vi "Write Position.vi"(8 "error in":errorcluster, 10 "Position":bool, 11 "Switch Step in":refnum<class "Switch Step.lvclass">) -> (0 "error out":errorcluster, 3 "Switch Step out":refnum<class "Switch Step.lvclass">)   [LabVIEW 2012, in "Sequence Composition.lvlib" / "Switch Step.lvclass"]
uses:
  Switch Step.lvclass
  Switch Step.lvclass/Switch Step.ctl
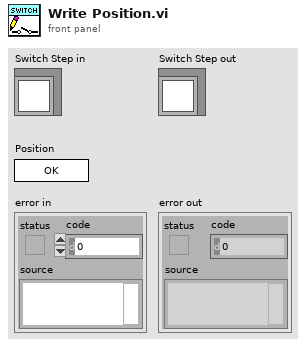
[diagram p1: front panel]
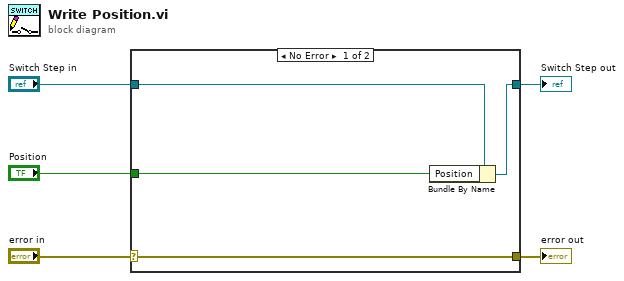
[diagram p0: block diagram]
diagram:
  n1 = case shown="No Error" "error in" {
    selector: "error in" -> [w9 w10]
    tunnel: [w9 w10] -> w4
    tunnel: [w7 w11] -> w2
    tunnel: "Switch Step in" -> [w8 w11]
    tunnel: "Position" -> [w6 _]
    frame No Error {
      n2 = Bundle By Name(cluster=w8, "Position"=w6) -> (w7:refnum<class "Switch Step.lvclass">)
    }
    frame Error {
    }
  }
  "error out" <- w4
  "Switch Step out" <- w2
